vi "MEMR-Read Data File.vi"(0 "Path":path=path "D:/Data/MEMR/Ken/SFMH41-MEMR-1.txt", 11 "Error In":errorcluster) -> (4 "Path (dup)":path=path "D:/Data/MEMR/Ken/SFMH41-MEMR-1.txt", 6 "Params":T1, 8 "IO":cluster{"Level":dbl[], "Gain":dbl[]}, 10 "Spectra":cluster{dbl[], dbl[][]}[](array[cluster]), 15 "error out":errorcluster)   [LabVIEW 2020]
uses:
  Typedefs/MEMR-Params.ctl
  Typedefs/MEMR-Probe.ctl
  Typedefs/MEMR-Elicitor.ctl
  Human Studies/SFM Frontend/LV Source/Typedefs/HSTS-Transducer.ctl
  Typedefs/MEMR-Sequence.ctl
  Typedefs/MEMR-Analysis.ctl
  Typedefs/MEMR-Timing.ctl
  <vilib>/regexp/Match Regular Expression.xnode
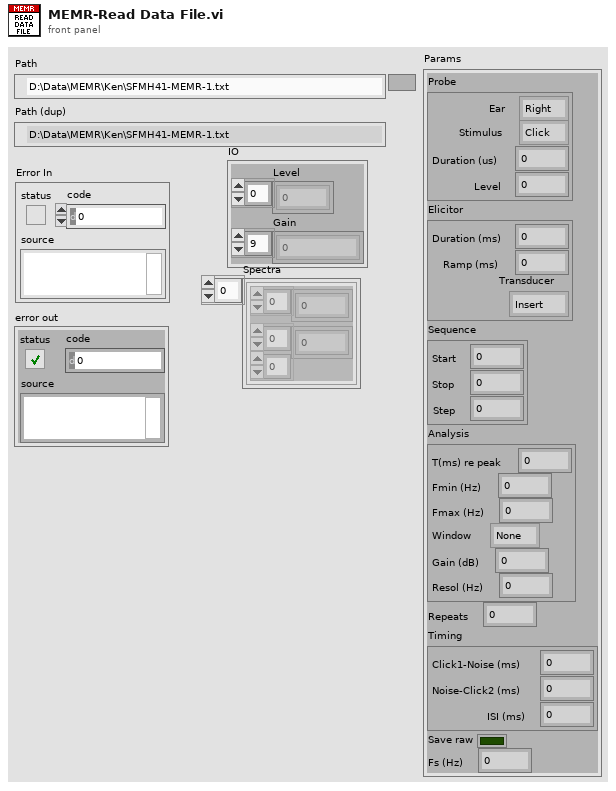
[diagram p1: front panel]
types:
  T1 = typedef "MEMR-Params.ctl" = cluster{"Probe":T2, "Elicitor":T3, "Sequence":T5, "Analysis":T6, "Repeats":i32, "Timing":T7, "Save raw":bool, "Fs (Hz)":dbl}
  T2 = typedef "MEMR-Probe.ctl" = cluster{"Ear":enum16{"Right", "Left"}, "Stimulus":enum16{"Click", "Chirp"}, "Duration (us)":dbl, "Level":dbl}
  T3 = typedef "MEMR-Elicitor.ctl" = cluster{"Duration (ms)":dbl, "Ramp (ms)":dbl, "Transducer":T4}
  T4 = typedef "HSTS-Transducer.ctl" = enum16{"Insert", "TDH-39", "HD300", "ER-10X"}
  T5 = typedef "MEMR-Sequence.ctl" = cluster{"Start":dbl, "Stop":dbl, "Step":dbl}
  T6 = typedef "MEMR-Analysis.ctl" = cluster{"T(ms) re peak":dbl, "Fmin (Hz)":dbl, "Fmax (Hz)":dbl, "Window":enum16{"None", "Hanning", "Hamming"}, "Gain (dB)":dbl, "Resol (Hz)":dbl}
  T7 = typedef "MEMR-Timing.ctl" = cluster{"Click1-Noise (ms)":dbl, "Noise-Click2 (ms)":dbl, "ISI (ms)":dbl}
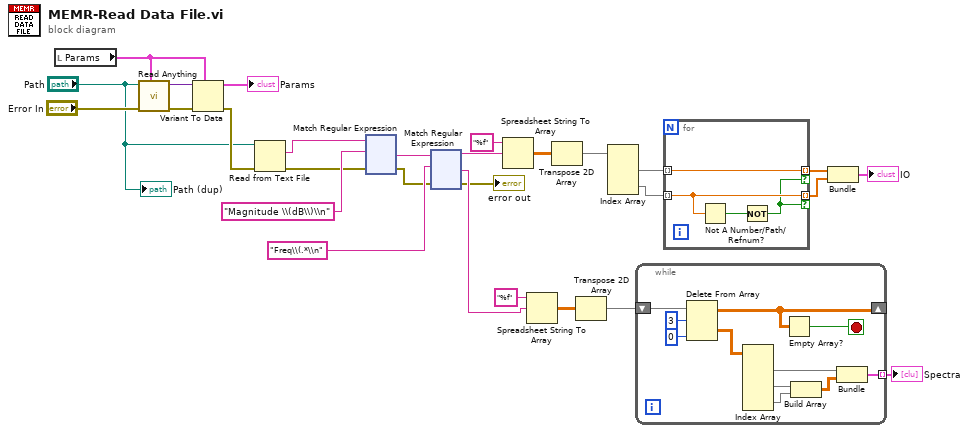
[diagram p0: block diagram]
diagram:
  n1 = local read "Params"() -> (w28:T1)
  n2 = call "Read Anything.vi"("Type of Anything"=w28, "Error In"="Error In", "Path (dialog)"="Path") -> ("Error Out"=w26:errorcluster, "Anything"=w27:variant)  [unwired: 6 in, 1 out]
  n3 = Variant To Data(error in=w26, type=w28, Variant=w27) -> (data=→"Params":T1, error out=w23:errorcluster)
  n4 = Read from Text File(file (use dialog)="Path", error in=w23) -> (text=w21:string, error out=w19:errorcluster)  [unwired: 2 in, 2 out]
  n5 = xnode "Match Regular Expression"("input string"=w21, "regular expression"="Magnitude \\(dB\\)\\n", "error in"=w19) -> ("after match"=w18:string, "error out"=w11:errorcluster)  [unwired: 3 in, 3 out]
  n6 = xnode "Match Regular Expression"("input string"=w18, "regular expression"="Freq\\(.*\\n", "error in"=w11) -> ("before match"=w16:string, "after match"=w8:string, "error out"=→"error out":errorcluster)  [unwired: 3 in, 2 out]
  n7 = Spreadsheet String To Array(format string="%f", spreadsheet string=w16) -> (array=w14:dbl[][])  [unwired: 2 in]
  n8 = Spreadsheet String To Array(format string="%f", spreadsheet string=w8) -> (array=w9:dbl[][])  [unwired: 2 in]
  n9 = Transpose 2D Array(2D array=w14) -> (transposed array=w13:dbl[][])
  n10 = Transpose 2D Array(2D array=w9) -> (transposed array=w6:dbl[][])
  n11 = Index Array(array=w13) -> (element #1=w1:dbl[], element #2=w4:dbl[])  [unwired: 4 in]
  n12 = while {
    shift-right: [w37] -> _
    shift-left: w6 -> [w39]
    tunnel: [w30] -> w5 mode=indexing
    stop <- w36 stop-if-true
    n13 = Delete From Array(array=w39, length=3, index (row)=0) -> (deleted portion=w35:dbl[][], array with subset deleted=w37:dbl[][])  [unwired: 1 in]
    n14 = Index Array(array=w35) -> (element #1=w34:dbl[], element #2=w33:dbl[], element #3=w32:dbl[])  [unwired: 6 in]
    n15 = Empty Array?(array=w37) -> (empty?=w36:bool)
    n16 = Build Array(w33, w32) -> (w31:dbl[][])
    n17 = Bundle(w34, w31) -> (w30:cluster{dbl[], dbl[][]})  [unwired: 1 in]
  }
  "Spectra" <- w5
  n18 = for {
    tunnel: w4 -> [w43] mode=indexing
    tunnel: [w43] -> w3 mode=indexing if=w40
    tunnel: [w42] -> w2 mode=indexing if=w40
    tunnel: w1 -> [w42] mode=indexing
    n19 = Not A Number/Path/Refnum?(number/path/refnum=w43) -> (NaN/Path/Refnum?=w41:bool)
    n20 = Not(x=w41) -> (.not. x?=w40:bool)
  }
  n21 = Bundle(w2, w3) -> (→"IO":cluster{dbl[], dbl[]})  [unwired: 1 in]
  "Path (dup)" <- "Path"
